vi "Gray's Lidar Tilt Excercize.vi"() -> ()   [LabVIEW 2009]
uses:
  <vilib>/userDefined/High Color/nirio_resource_hc.ctl
  Strict Lidar Motor Control Cluster.ctl
  Strict Lidar Motor Indicator Cluster.ctl
  <vilib>/rvi/interface/nirviOpenFPGA/nirviOpenFPGA.xnode
  FPGA Bitfiles/Athena Brain.lvproj_FPGA Target 2_Gray's Mod Motor C~4B.lvbitx
  <vilib>/FPGAPlugInAG/sbRIO-9642/nirviIntfOpen_sbRIO-9642.vi
  <vilib>/rvi/interface/nirviReadWriteControl/nirviReadWriteControl.xnode
  <vilib>/LabVIEW Targets/FPGA/RIO/nirio_HostInterface/nirio_WriteBig.vi
  <vilib>/LabVIEW Targets/FPGA/RIO/nirio_HostInterface/nirio_ReadBig.vi
  <vilib>/Utility/error.llb/Error Cluster From Error Code.vi
  <vilib>/rvi/errors/niLvFpgaAdjustHostInterfaceError.vi
  <vilib>/rvi/interface/common/niFpgaNodeNameForErrorReporting.ctl
  <vilib>/rvi/errors/niLvFpgaWhatHappensToTopLevelVI.ctl
  NiRioSrv.dll
panel:
  out "Lidar Encoder":i32
  out "Error 32b int (enc)":i32
  in  "Count(uSec) 2":u32 caption="Count(uSec)"
  out "output cluster":T1 {"?"."D Error" format="%.18g"; "?"."D portion" format="%.18g"; "?"."DD Error" format="%.18g"; "?"."DD portion" format="%.18g"; "?"."I Error" format="%.18g"; "?"."I portion" format="%.18g"; "?"."II Error" format="%.18g"; "?"."II portion" format="%.18g"; "?"."P Error" format="%.18g"; "?"."P portion" format="%.18g"}
  out "setpoint":i32
  in  "osc mag":dbl
  in  "osc offset":dbl
  out "x+1":i8
  in  "Count(uSec)":u32
  out "Server 1 Timeouts by Identifier":bool[](array[boolean])
  out "Lidar Motor Indicator":T2
  in  "Lidar Motor Control":T3={"Reset Encoder"=FALSE, "Motor Enable"=FALSE, "Choice of Control Type"=enum."Direct Voltage Control", "Choice of Oscillation"=enum."Oscillate Voltage", "Choice of Compensation"=enum."None", "Choice of Error"=enum."Gray Error", "Units of pi rad 18b (s-fxp-1)"={"Phi_B Set Point (pi rad)"=0.0, "Phi_A Set Point (pi rad)"=0.0, "Phi_Lidar Set Point (pi rad)"=0.0, "Phi_Lidar - Phi_A"=0.0, "Phi_mass-Phi_Lidar"=0.0, "Convert (enc) to (pi rad)"=0.0, "Oscillation Frequency (pi rad per 100KHz)"=0.0}, "Units of 18b (s-fxp-1) gain"={"Proportional Gain"=0.0, " Integral Gain"=0.0, "Oscillation Setpoint Amplitude"=0.0, "Gravity Compensation Gain"=0.0, "Phi_B Set Point (enc) pre-gain"=0.0, "Phi_B Set Point (pi rad) pre-gain"=0.0, "Phi_A Set Point (pi rad) pre-gain"=0.0, "Phi_Lidar Set Point (pi rad) pre-gain"=0.0, "Derivative Gain"=0.0, "Double Integral Gain"=0.0, "Second Derivative Gain"=0.0}, "Units of 20b s-fxp-5 Voltage"={"Oscillation Voltage Amplitude"=0.0, "Motor Voltage"=0.0}, "Units of encoder 32b uint"={"Phi_B Set Point (enc)"=0, "Lidar Encoder Cap"=0}, "Debug Args"=[FALSE, FALSE, FALSE, FALSE, FALSE, FALSE, FALSE, FALSE, FALSE, FALSE, FALSE, FALSE, FALSE, FALSE, FALSE, FALSE, FALSE, FALSE, FALSE, FALSE], "Units of 8b int gain exponents"={"Proportional Gain"=0, " Integral Gain"=0, "Oscillation Setpoint Amplitude"=0, "Gravity Compensation Gain"=0, "Phi_B Set Point (enc) pre-gain"=0, "Phi_B Set Point (pi rad) pre-gain"=0, "Phi_A Set Point (pi rad) pre-gain"=0, "Phi_Lidar Set Point (pi rad) pre-gain"=0, "Derivative Gain"=0, "Double Integral Gain"=0, "Second Derivative Gain"=0}, "6b (u-fxp-6)"={"Size of Integrator"=0.0, "Size of IIntigrator"=0.0, "Size of Differentiator"=0.0, "Size of DDifferentiator"=0.0}} {"Units of 20b s-fxp-5 Voltage"."Motor Voltage" format="%.17g"}
  in  "stop":bool
  in  "RIO Device":T4
  # "50Hz Update Frequency"
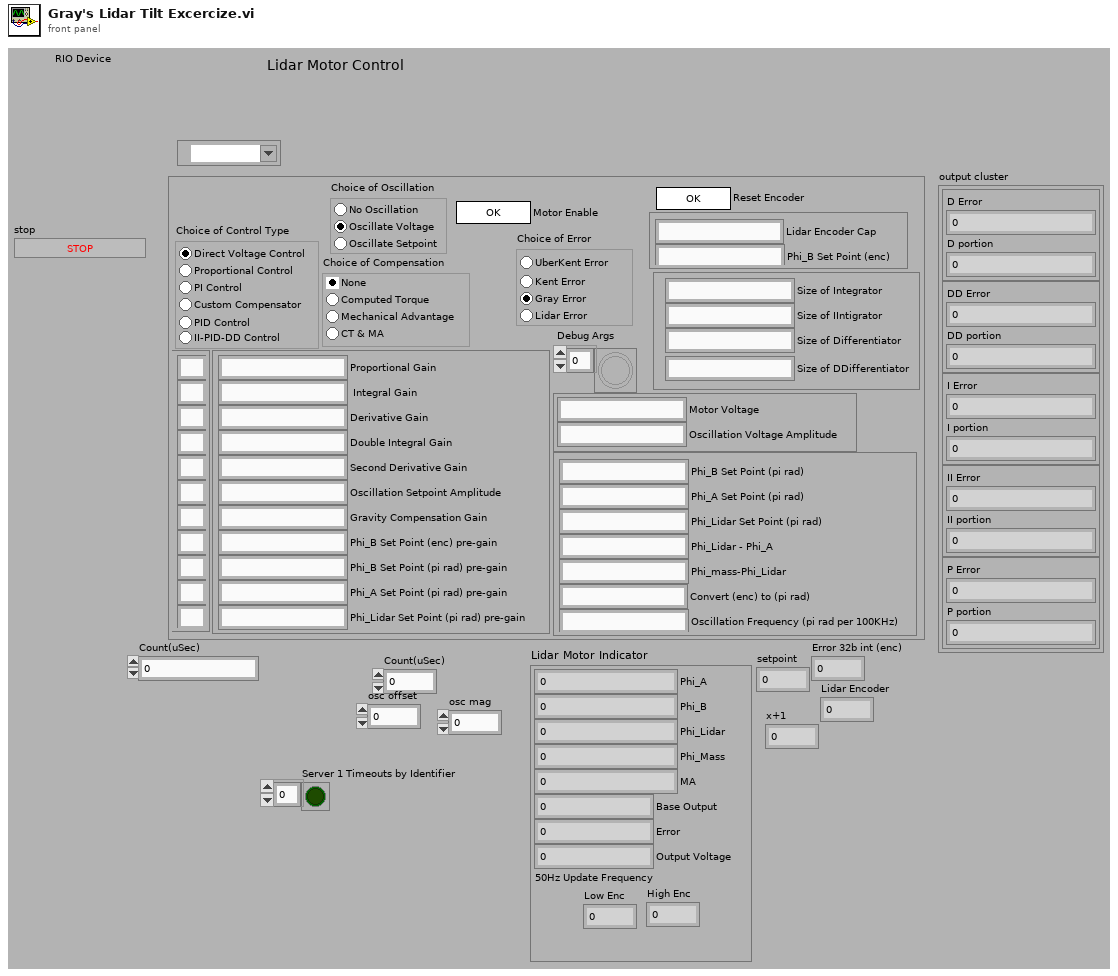
[diagram p1: front panel]
types:
  T1 = cluster{cluster{"D Error":fxp<+/-,18,1>, "D portion":fxp<+/-,18,1>}, cluster{"DD Error":fxp<+/-,18,1>, "DD portion":fxp<+/-,18,1>}, cluster{"I Error":fxp<+/-,18,1>, "I portion":fxp<+/-,18,1>}, cluster{"II Error":fxp<+/-,18,1>, "II portion":fxp<+/-,18,1>}, cluster{"P Error":fxp<+/-,18,1>, "P portion":fxp<+/-,18,1>}}
  T2 = typedef "Strict Lidar Motor Indicator Cluster.ctl" = cluster{"Phi_A":fxp<+/-,18,1>, "Phi_B":fxp<+/-,18,1>, "Output Voltage":fxp<+/-,20,5>, "Phi_Lidar":fxp<+/-,18,1>, "Phi_Mass":fxp<+/-,18,1>, "MA":fxp<+/-,18,1>, "Base Output":fxp<+/-,18,1>, "Error":fxp<+/-,18,1>, "Low Enc":i32, "High Enc":i32}
  T3 = typedef "Strict Lidar Motor Control Cluster.ctl" = cluster{"Reset Encoder":bool, "Motor Enable":bool, "Choice of Control Type":enum32{"Direct Voltage Control", "Proportional Control", "PI Control", "Custom Compensator", "PID Control", "II-PID-DD Control"}, "Choice of Oscillation":enum32{"Oscillate Voltage", "Oscillate Setpoint", "No Oscillation"}, "Choice of Compensation":enum32{"None", "Computed Torque", "Mechanical Advantage", "CT & MA "}, "Choice of Error":enum32{"Gray Error", "Lidar Error", "Kent Error", "UberKent Error"}, "Units of pi rad 18b (s-fxp-1)":cluster{"Phi_B Set Point (pi rad)":fxp<+/-,18,1>, "Phi_A Set Point (pi rad)":fxp<+/-,18,1>, "Phi_Lidar Set Point (pi rad)":fxp<+/-,18,1>, "Phi_Lidar - Phi_A":fxp<+/-,18,1>, "Phi_mass-Phi_Lidar":fxp<+/-,18,1>, "Convert (enc) to (pi rad)":fxp<+/-,18,1>, "Oscillation Frequency (pi rad per 100KHz)":fxp<+/-,18,1>}, "Units of 18b (s-fxp-1) gain":cluster{"Proportional Gain":fxp<+/-,18,1>, " Integral Gain":fxp<+/-,18,1>, "Oscillation Setpoint Amplitude":fxp<+/-,18,1>, "Gravity Compensation Gain":fxp<+/-,18,1>, "Phi_B Set Point (enc) pre-gain":fxp<+/-,18,1>, "Phi_B Set Point (pi rad) pre-gain":fxp<+/-,18,1>, "Phi_A Set Point (pi rad) pre-gain":fxp<+/-,18,1>, "Phi_Lidar Set Point (pi rad) pre-gain":fxp<+/-,18,1>, "Derivative Gain":fxp<+/-,18,1>, "Double Integral Gain":fxp<+/-,18,1>, "Second Derivative Gain":fxp<+/-,18,1>}, "Units of 20b s-fxp-5 Voltage":cluster{"Oscillation Voltage Amplitude":fxp<+/-,20,5>, "Motor Voltage":fxp<+/-,20,5>}, "Units of encoder 32b uint":cluster{"Phi_B Set Point (enc)":i32, "Lidar Encoder Cap":i32}, "Debug Args":bool[], "Units of 8b int gain exponents":cluster{"Proportional Gain":i8, " Integral Gain":i8, "Oscillation Setpoint Amplitude":i8, "Gravity Compensation Gain":i8, "Phi_B Set Point (enc) pre-gain":i8, "Phi_B Set Point (pi rad) pre-gain":i8, "Phi_A Set Point (pi rad) pre-gain":i8, "Phi_Lidar Set Point (pi rad) pre-gain":i8, "Derivative Gain":i8, "Double Integral Gain":i8, "Second Derivative Gain":i8}, "6b (u-fxp-6)":cluster{"Size of Integrator":fxp<+,6,6>, "Size of IIntigrator":fxp<+,6,6>, "Size of Differentiator":fxp<+,6,6>, "Size of DDifferentiator":fxp<+,6,6>}}
  T4 = typedef "nirio_resource_hc.ctl" = tag
  T5 = typedef "niFpgaNodeNameForErrorReporting.ctl" = enum16{"Open FPGA VI Reference", "Read/Write Control", "Invoke Method: Abort", "Invoke Method: Acknowledge IRQ", "Invoke Method: Download", "Invoke Method: FIFO.Configure", "Invoke Method: FIFO.Read", "Invoke Method: FIFO.Start", "Invoke Method: FIFO.Stop", "Invoke Method: FIFO.Write", "Invoke Method: Reset", "Invoke Method: Run", "Invoke Method: Wait on IRQ", "Close FPGA VI Reference"}
  T6 = typedef "niLvFpgaWhatHappensToTopLevelVI.ctl" = enum16{"top level VI scripted behind XNode", "top level VI inlined behind XNode"}
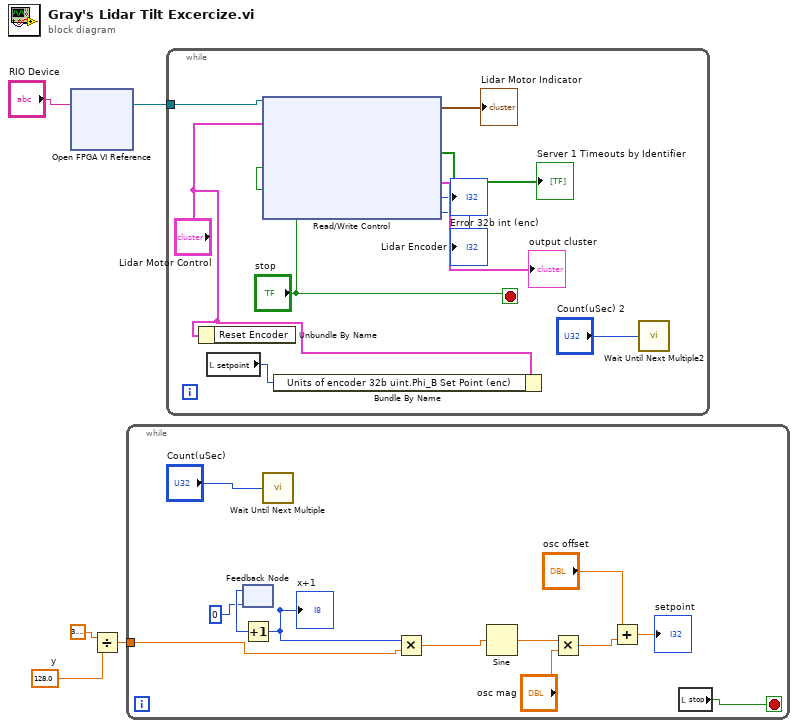
[diagram p0: block diagram]
diagram:
  w2 = 128.0  # y
  n1 = xnode "Open FPGA VI Reference"("resource name"="RIO Device") -> ("FPGA VI Reference Out"=w4:refnum<k20>)  [unwired: 1 in, 1 out]
  n2 = Divide(x=3.141592653589793, y=w2) -> (x/y=w1:dbl)
  n3 = while {
    tunnel: w1 -> [w14]
    stop <- w6 stop-if-true
    n4 = feedback #1(i8 0) -> (w16:i8)
    n5 = Increment(x=w16) -> (x+1=w13:i8)
    "x+1" <- w13
    n6 = call "Wait Until Next Multiple"("Count(uSec)"="Count(uSec)") -> ()  [unwired: 1 out]
    n7 = Multiply(x=w13, y=w14) -> (x*y=w12:dbl)
    n8 = Sine(x=w12) -> (sin(x)=w11:dbl)
    n9 = Multiply(x=w11, y="osc mag") -> (x*y=w10:dbl)
    n10 = Add(x="osc offset", y=w10) -> (x+y=→"setpoint":dbl)
    n11 = local read "stop"() -> (w6:bool)
  }
  n12 = while {
    tunnel: w4 -> [w27]
    stop <- "stop" stop-if-true
    n13 = Unbundle By Name("Lidar Motor Control") -> ()  [unwired: 1 out]
    n14 = local read "setpoint"() -> (w22:i32)
    n15 = xnode "Read/Write Control"("FPGA VI Reference In"=w27, "Lidar Motor Control"="Lidar Motor Control", "Stop"="stop") -> ("Lidar Motor Indicator"=→"Lidar Motor Indicator":T2, "Server 1 Timeouts by Identifier"=→"Server 1 Timeouts by Identifier":bool[], "output cluster"=→"output cluster":T1, "Error 32b int (enc)"=→"Error 32b int (enc)":i32, "Lidar Encoder"=→"Lidar Encoder":i32)  [unwired: 1 in, 2 out]
    n16 = Bundle By Name(cluster="Lidar Motor Control", "Units of encoder 32b uint.Phi_B Set Point (enc)"=w22) -> ()  [unwired: 1 out]
    n17 = call "Wait Until Next Multiple2"("Count(uSec)"="Count(uSec) 2") -> ()  [unwired: 1 out]
  }
